vi "Analyze Read.vi"(0 "VISA in":refnum<visa-resource-name>, 1 "String":string, 3 "error in (no error)":errorcluster) -> (7 "VISA out":refnum<visa-resource-name>, 8 "Stop?":bool, 10 "error out":errorcluster)   [LabVIEW 2017]
panel:
  out "Error Array Size":dbl
  out "CLR":u32
  out "MAMP":u32
  out "Prta Number":string
  out "Prts Number":string
  out "BLD":u32
  out "EE ROM":string
  out "Array Size":i32
  out "Part Number":string
  out "VBUS":u32
  out "EERD":u32 format="%.0x"
  out "LOOP":u32 format="%.0x"
  out "LFTG":u32
  out "LFTS":u32
  out "LIFT":u32
  out "BRK":u32
  out "RPMH":u32
  out "RPML":u32
  out "PRPM":u32
  out "REV":u32
  out "RPM":u32
  out "SECS":u32
  out "ACAD":u32
  out "BATL":u32
  out "BATC":u32
  out "VCHG":u32
  out "VBAT":u32
  out "RES":u32
  out "RAMP":u32
  out "Error Codes":u8[](array[numeric])
  out "Array":string[](array[string])
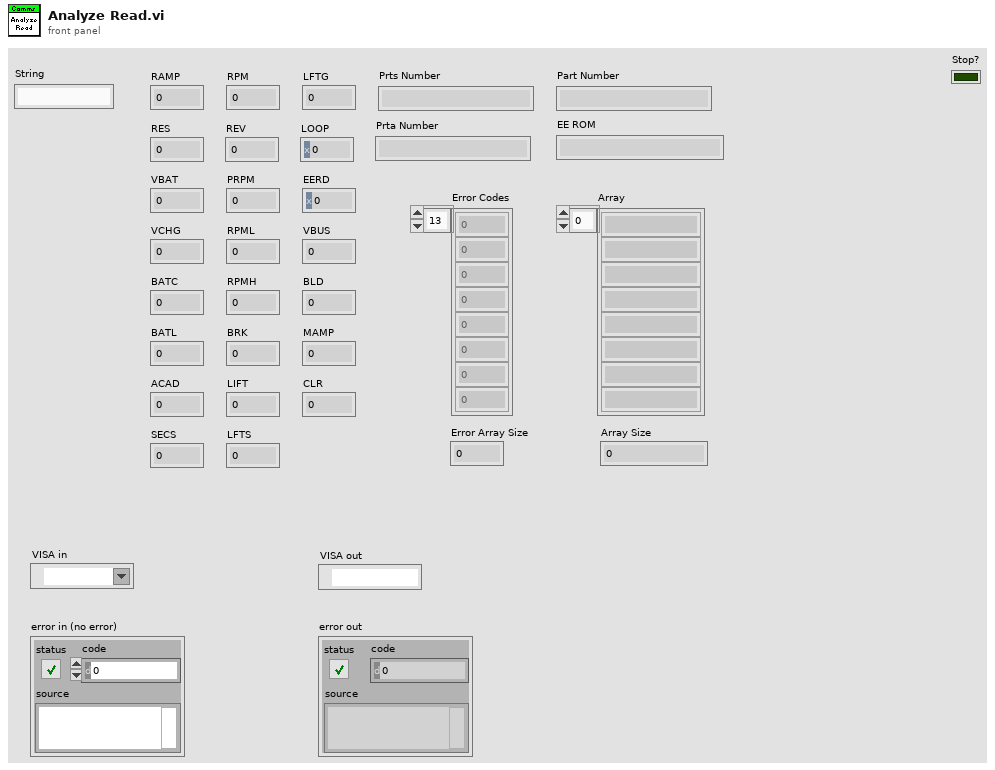
[diagram p1: front panel]
types:
  T1 = enum16{"Init", "Get Index", "Analyze Part", "Analyze Prts", "Analyze Prta", "Set VER", "Set TYPE"}
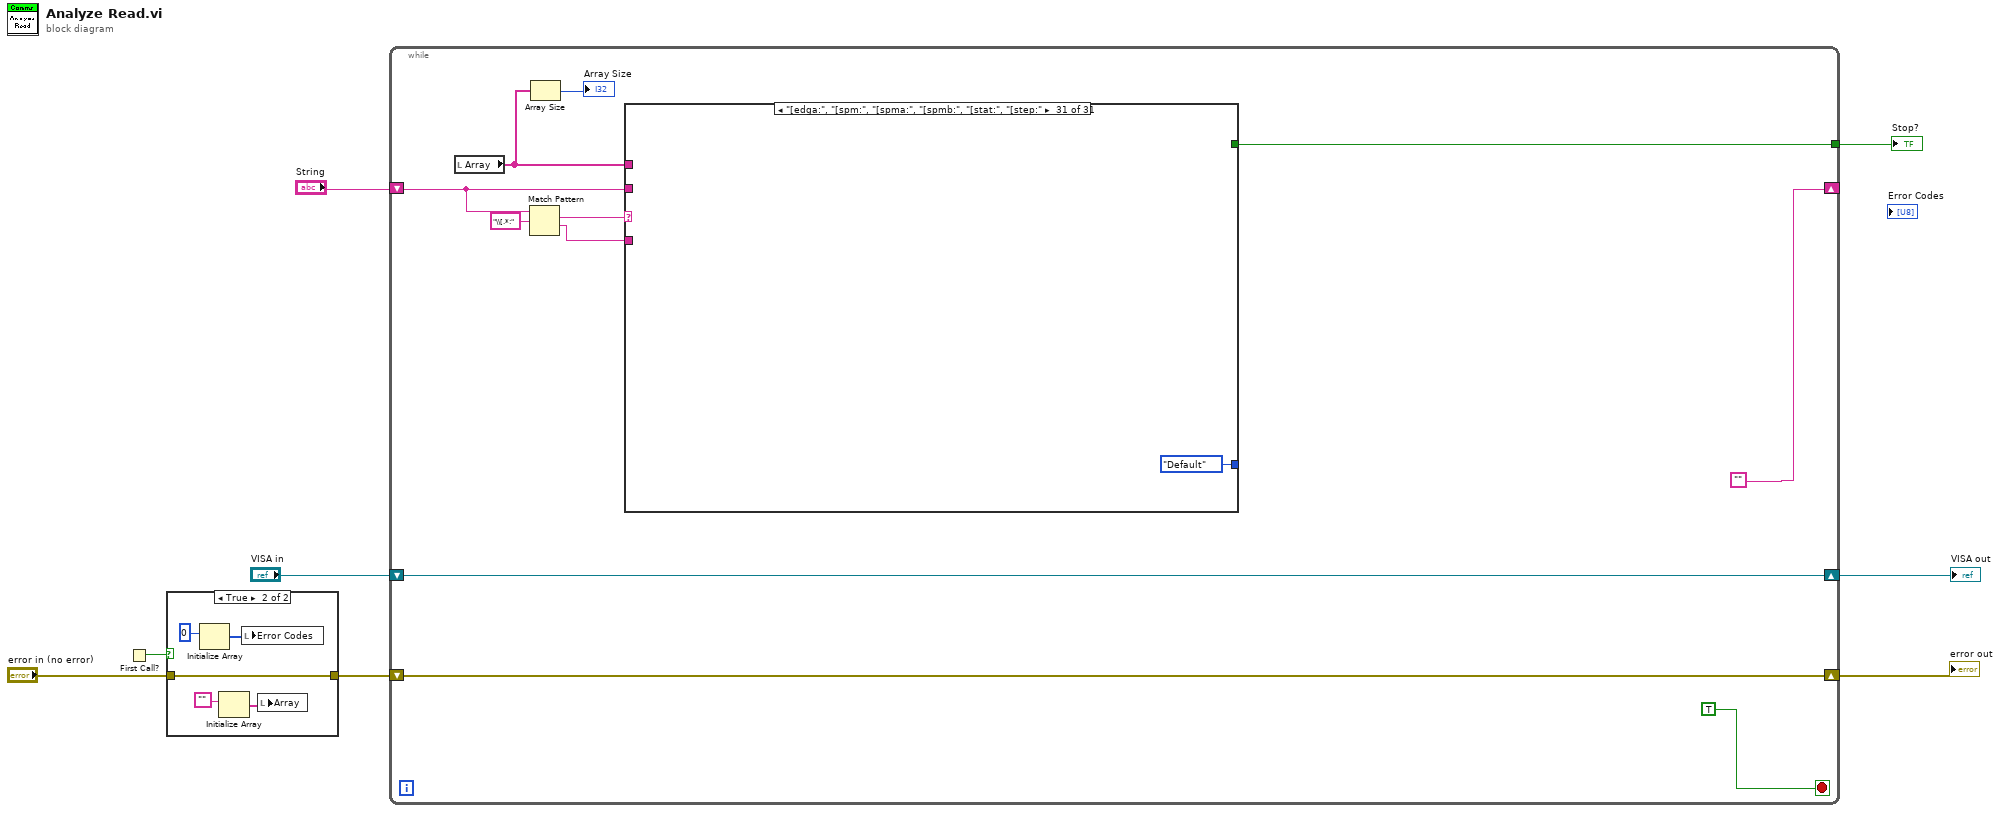
[diagram p0: block diagram]
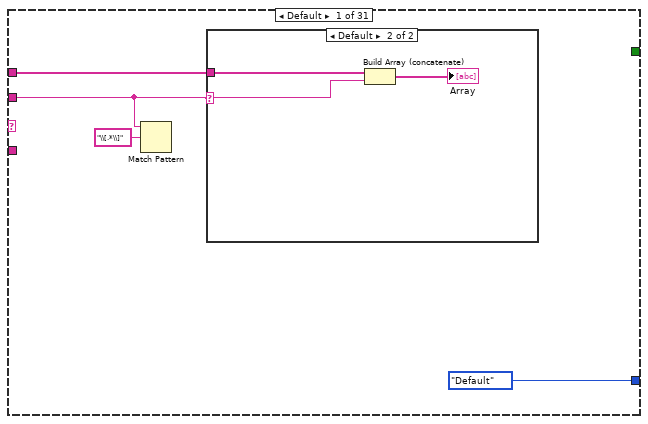
[diagram p3: hidden frame]
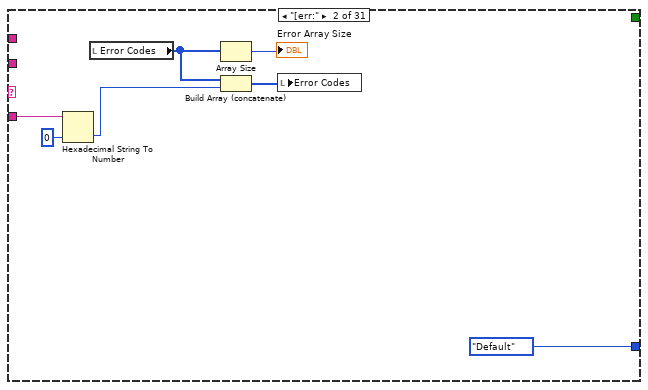
[diagram p5: hidden frame]
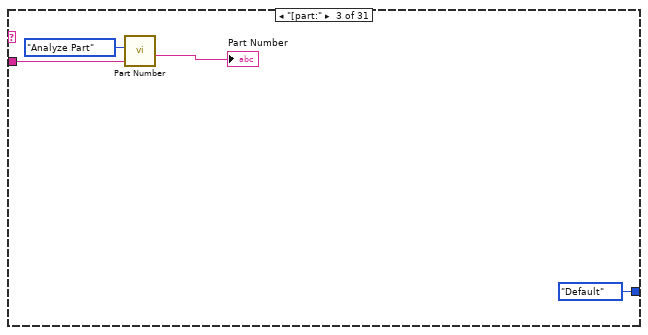
[diagram p6: hidden frame]
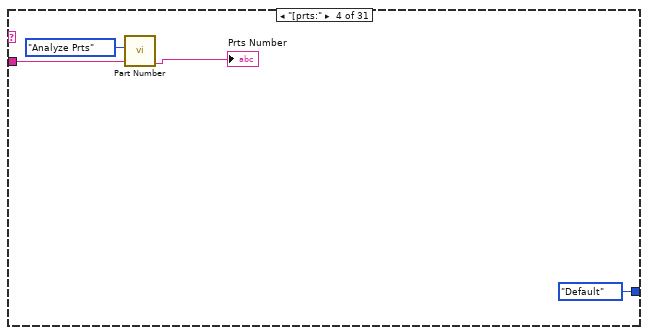
[diagram p7: hidden frame]
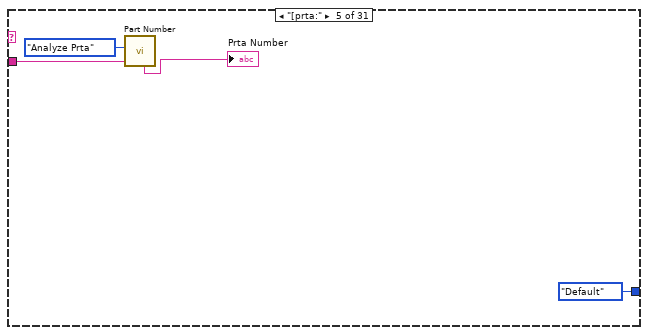
[diagram p8: hidden frame]
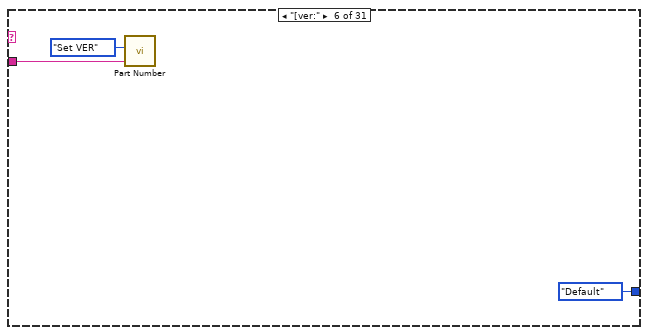
[diagram p9: hidden frame]
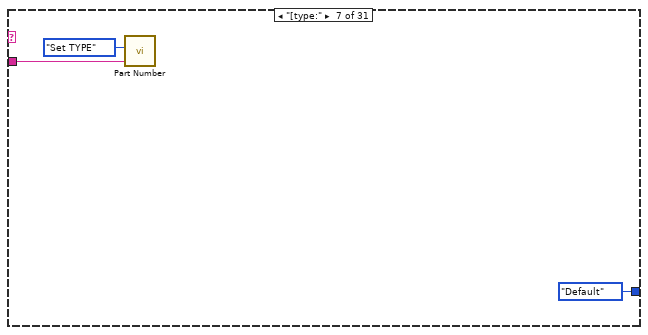
[diagram p10: hidden frame]
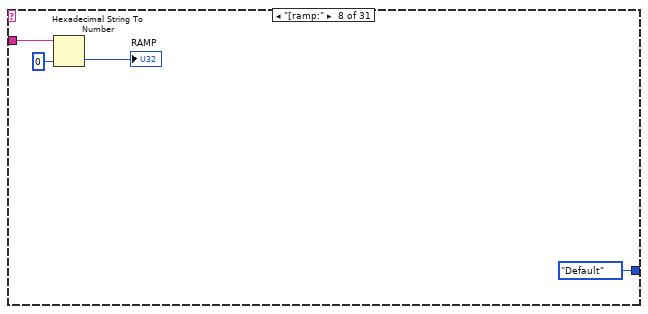
[diagram p11: hidden frame]
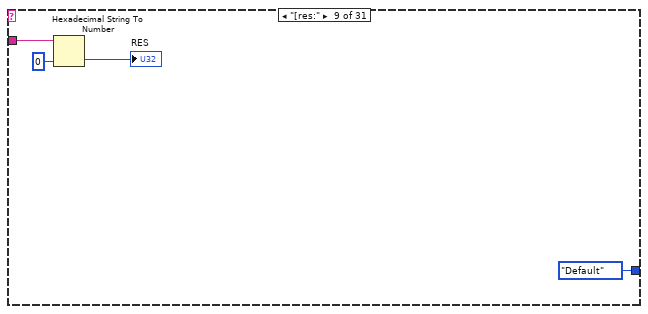
[diagram p12: hidden frame]
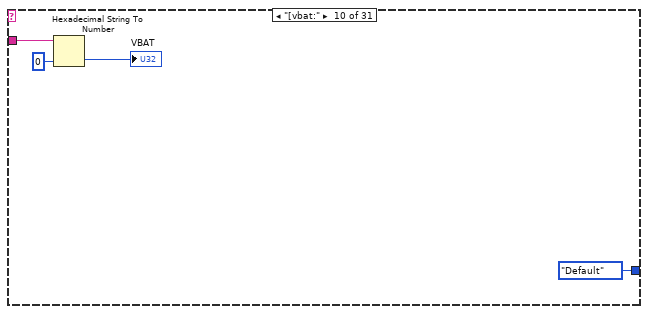
[diagram p13: hidden frame]
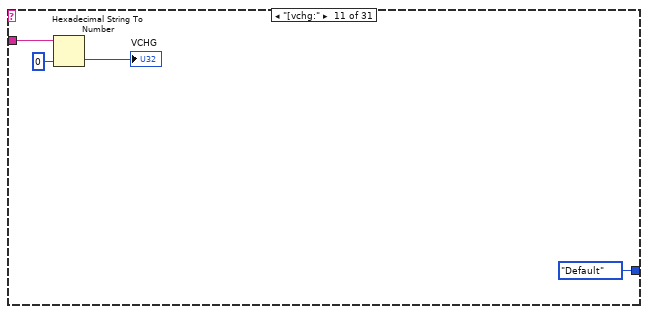
[diagram p14: hidden frame]
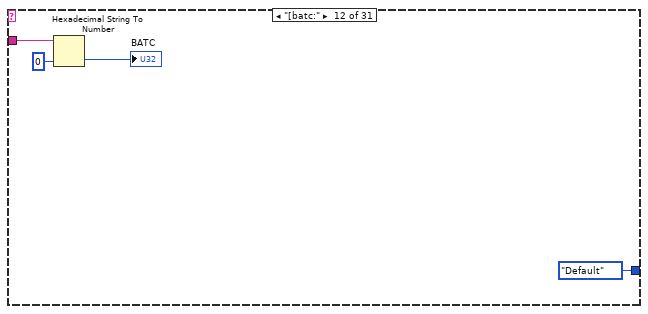
[diagram p15: hidden frame]
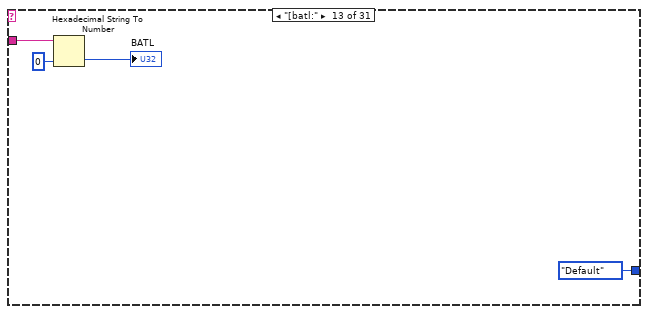
[diagram p16: hidden frame]
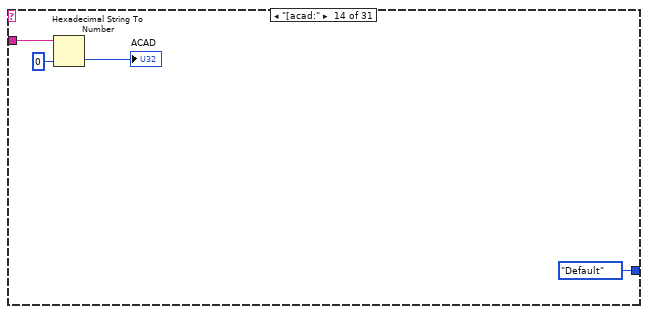
[diagram p17: hidden frame]
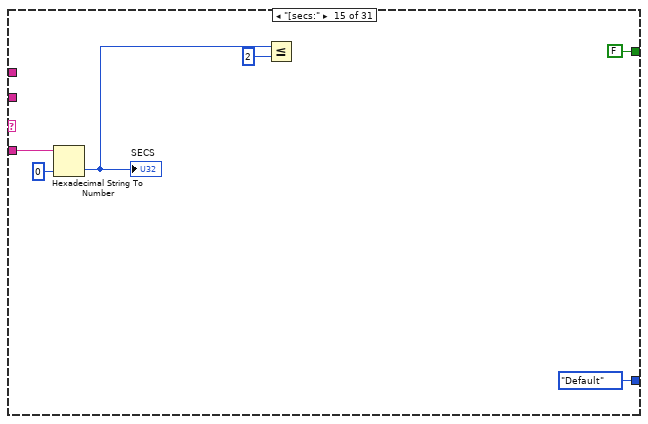
[diagram p18: hidden frame]
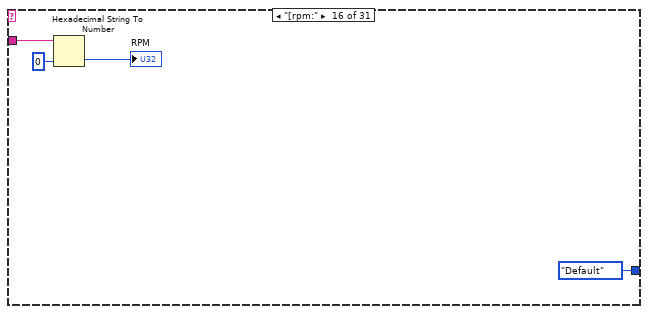
[diagram p19: hidden frame]
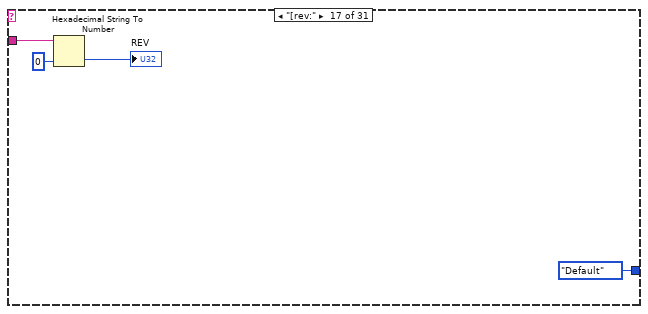
[diagram p20: hidden frame]
diagram:
  n1 = First Call?() -> (First Call?: T/F=w1:bool)
  n2 = case shown="True" w1 {
    tunnel: "error in (no error)" -> [w9 w14]
    tunnel: [w9 w14] -> w2
    frame False {
    }
    frame True {
      n3 = Initialize Array(0) -> (w11:i32[])  [unwired: 1 in]
      n4 = Initialize Array("") -> (w13:string[])  [unwired: 1 in]
      n5 = local write "Error Codes"(w11) -> ()
      n6 = local write "Array"(w13) -> ()
    }
  }
  n7 = while {
    shift-right: [w21] -> w6
    shift-left: "VISA in" -> [w21]
    shift-right: [w20] -> w5
    shift-left: w2 -> [w20]
    shift-right: [""] -> _
    shift-left: "String" -> [w22]
    tunnel: [w15] -> w4
    stop <- TRUE stop-if-true
    n8 = local read "Array"() -> (w16:string[])
    n9 = Match Pattern(string=w22, regular expression="\\[.*:") -> (match substring=w24:string, after substring=w23:string)  [unwired: 1 in, 2 out]
    n10 = Array Size(array=w16) -> (size(s)=→"Array Size":i32)
    n11 = case shown="\"[edga:\", \"[spm:\", \"[spma:\", \"[spmb:\", \"[stat:\", \"[step:\"" w24 {
      tunnel: w23 -> [_ w38 w42 w46 w50 w53 w56 w60 w64 w68 w72 w76 w80 w84 w90 w94 w98 w102 w106 w110 w114 w118 w122 w126 w130 w134 w140 w144 w148 w152 _]
      tunnel: w22 -> [w27 _ _ _ _ _ _ _ _ _ _ _ _ _ _ _ _ _ _ _ _ _ _ _ _ _ _ _ _ _ _]
      tunnel: [enum16{"Default", "Send RSET"}."Default" enum16{"Default", "Send RSET"}."Default" enum16{"Default", "Send RSET"}."Default" enum16{"Default", "Send RSET"}."Default" enum16{"Default", "Send RSET"}."Default" enum16{"Default", "Send RSET"}."Default" enum16{"Default", "Send RSET"}."Default" enum16{"Default", "Send RSET"}."Default" enum16{"Default", "Send RSET"}."Default" enum16{"Default", "Send RSET"}."Default" enum16{"Default", "Send RSET"}."Default" enum16{"Default", "Send RSET"}."Default" enum16{"Default", "Send RSET"}."Default" enum16{"Default", "Send RSET"}."Default" enum16{"Default", "Send RSET"}."Default" enum16{"Default", "Send RSET"}."Default" enum16{"Default", "Send RSET"}."Default" enum16{"Default", "Send RSET"}."Default" enum16{"Default", "Send RSET"}."Default" enum16{"Default", "Send RSET"}."Default" enum16{"Default", "Send RSET"}."Default" enum16{"Default", "Send RSET"}."Default" enum16{"Default", "Send RSET"}."Default" enum16{"Default", "Send RSET"}."Default" enum16{"Default", "Send RSET"}."Default" enum16{"Default", "Send RSET"}."Default" enum16{"Default", "Send RSET"}."Default" enum16{"Default", "Send RSET"}."Default" enum16{"Default", "Send RSET"}."Default" enum16{"Default", "Send RSET"}."Default" enum16{"Default", "Send RSET"}."Default"] -> _
      tunnel: w16 -> [w26 _ _ _ _ _ _ _ _ _ _ _ _ _ _ _ _ _ _ _ _ _ _ _ _ _ _ _ _ _ _]
      tunnel: [_ _ _ _ _ _ _ _ _ _ _ _ _ _ FALSE _ _ _ _ _ _ _ _ _ _ _ _ _ _ _ _] -> w15
      frame Default {
        n12 = Match Pattern(string=w27, regular expression="\\[.*\\]") -> ()  [unwired: 1 in, 4 out]
        n13 = case shown="Default" w27 {
          selector: w27 -> [_ w32]
          tunnel: w26 -> [_ w31]
          frame "[err]" {
          }
          frame Default {
            n14 = Build Array (concatenate)(w31, w32) -> (→"Array":string[])
          }
        }
      }
      frame "[err:" {
        n15 = Hexadecimal String To Number(string=w38, default (0uL)=u8 0 ("default (0 U32)")) -> (number=w36:u8)  [unwired: 1 in, 1 out]
        n16 = local read "Error Codes"() -> (w34:u8[])
        n17 = Array Size(array=w34) -> (size(s)=→"Error Array Size":i32)
        n18 = Build Array (concatenate)(w34, w36) -> (w37:u8[])
        n19 = local write "Error Codes"(w37) -> ()
      }
      frame "[part:" {
        n20 = call "Part Number.vi"("Value from LPCA"=w42, "Command"=T1."Analyze Part") -> ("Part Number"=→"Part Number":string)  [unwired: 4 in, 5 out]
      }
      frame "[prts:" {
        n21 = call "Part Number.vi"("Value from LPCA"=w46, "Command"=T1."Analyze Prts") -> ("Prts Number"=→"Prts Number":string)  [unwired: 4 in, 5 out]
      }
      frame "[prta:" {
        n22 = call "Part Number.vi"("Value from LPCA"=w50, "Command"=T1."Analyze Prta") -> ("Prta Number"=→"Prta Number":string)  [unwired: 4 in, 5 out]
      }
      frame "[ver:" {
        n23 = call "Part Number.vi"("Value from LPCA"=w53, "Command"=T1."Set VER") -> ()  [unwired: 4 in, 6 out]
      }
      frame "[type:" {
        n24 = call "Part Number.vi"("Value from LPCA"=w56, "Command"=T1."Set TYPE") -> ()  [unwired: 4 in, 6 out]
      }
      frame "[ramp:" {
        n25 = Hexadecimal String To Number(string=w60, default (0uL)=u32 0 ("default (0 U32)")) -> (number=→"RAMP":u32)  [unwired: 1 in, 1 out]
      }
      frame "[res:" {
        n26 = Hexadecimal String To Number(string=w64, default (0uL)=u32 0 ("default (0 U32)")) -> (number=→"RES":u32)  [unwired: 1 in, 1 out]
      }
      frame "[vbat:" {
        n27 = Hexadecimal String To Number(string=w68, default (0uL)=u32 0 ("default (0 U32)")) -> (number=→"VBAT":u32)  [unwired: 1 in, 1 out]
      }
      frame "[vchg:" {
        n28 = Hexadecimal String To Number(string=w72, default (0uL)=u32 0 ("default (0 U32)")) -> (number=→"VCHG":u32)  [unwired: 1 in, 1 out]
      }
      frame "[batc:" {
        n29 = Hexadecimal String To Number(string=w76, default (0uL)=u32 0 ("default (0 U32)")) -> (number=→"BATC":u32)  [unwired: 1 in, 1 out]
      }
      frame "[batl:" {
        n30 = Hexadecimal String To Number(string=w80, default (0uL)=u32 0 ("default (0 U32)")) -> (number=→"BATL":u32)  [unwired: 1 in, 1 out]
      }
      frame "[acad:" {
        n31 = Hexadecimal String To Number(string=w84, default (0uL)=u32 0 ("default (0 U32)")) -> (number=→"ACAD":u32)  [unwired: 1 in, 1 out]
      }
      frame "[secs:" {
        n32 = Hexadecimal String To Number(string=w90, default (0uL)=u32 0 ("default (0 U32)")) -> (number=w88:u32)  [unwired: 1 in, 1 out]
        "SECS" <- w88
        n33 = Less Or Equal?(x=w88, y=u32 2) -> ()  [unwired: 1 out]
      }
      frame "[rpm:" {
        n34 = Hexadecimal String To Number(string=w94, default (0uL)=u32 0 ("default (0 U32)")) -> (number=→"RPM":u32)  [unwired: 1 in, 1 out]
      }
      frame "[rev:" {
        n35 = Hexadecimal String To Number(string=w98, default (0uL)=u32 0 ("default (0 U32)")) -> (number=→"REV":u32)  [unwired: 1 in, 1 out]
      }
      frame "[prpm:" {
        n36 = Hexadecimal String To Number(string=w102, default (0uL)=u32 0 ("default (0 U32)")) -> (number=→"PRPM":u32)  [unwired: 1 in, 1 out]
      }
      frame "[rpml:" {
        n37 = Hexadecimal String To Number(string=w106, default (0uL)=u32 0 ("default (0 U32)")) -> (number=→"RPML":u32)  [unwired: 1 in, 1 out]
      }
      frame "[rpmh:" {
        n38 = Hexadecimal String To Number(string=w110, default (0uL)=u32 0 ("default (0 U32)")) -> (number=→"RPMH":u32)  [unwired: 1 in, 1 out]
      }
      frame "[brk:" {
        n39 = Hexadecimal String To Number(string=w114, default (0uL)=u32 0 ("default (0 U32)")) -> (number=→"BRK":u32)  [unwired: 1 in, 1 out]
      }
      frame "[lift:" {
        n40 = Hexadecimal String To Number(string=w118, default (0uL)=u32 0 ("default (0 U32)")) -> (number=→"LIFT":u32)  [unwired: 1 in, 1 out]
      }
      frame "[lfts:" {
        n41 = Hexadecimal String To Number(string=w122, default (0uL)=u32 0 ("default (0 U32)")) -> (number=→"LFTS":u32)  [unwired: 1 in, 1 out]
      }
      frame "[lftg:" {
        n42 = Hexadecimal String To Number(string=w126, default (0uL)=u32 0 ("default (0 U32)")) -> (number=→"LFTG":u32)  [unwired: 1 in, 1 out]
      }
      frame "[loop:" {
        n43 = Hexadecimal String To Number(string=w130, default (0uL)=u32 0 ("default (0 U32)")) -> (number=→"LOOP":u32)  [unwired: 1 in, 1 out]
      }
      frame "[eerd:" {
        n44 = Hexadecimal String To Number(string=w134, default (0uL)=u32 0 ("default (0 U32)")) -> (number=→"EERD":u32)  [unwired: 1 in, 1 out]
        n45 = call "ROM Data.vi"("Value from LPCA"=w134, "Command"=enum16{"Init", "Get Index", "Analyze"}."Analyze") -> ("ROM Data"=→"EE ROM":string)  [unwired: 1 out]
      }
      frame "[vbus:" {
        n46 = Hexadecimal String To Number(string=w140, default (0uL)=u32 0 ("default (0 U32)")) -> (number=→"VBUS":u32)  [unwired: 1 in, 1 out]
      }
      frame "[bld:" {
        n47 = Hexadecimal String To Number(string=w144, default (0uL)=u32 0 ("default (0 U32)")) -> (number=→"BLD":u32)  [unwired: 1 in, 1 out]
      }
      frame "[mamp:" {
        n48 = Hexadecimal String To Number(string=w148, default (0uL)=u32 0 ("default (0 U32)")) -> (number=→"MAMP":u32)  [unwired: 1 in, 1 out]
      }
      frame "[clr:" {
        n49 = Hexadecimal String To Number(string=w152, default (0uL)=u32 0 ("default (0 U32)")) -> (number=→"CLR":u32)  [unwired: 1 in, 1 out]
      }
      frame "[edga:", "[spm:", "[spma:", "[spmb:", "[stat:", "[step:" {
      }
    }
  }
  "error out" <- w5
  "VISA out" <- w6
  "Stop?" <- w4
